vi "Format Tablet Column Span.vi"(7 "Column Count":i32=1, 11 "Spanned Cell Text":string) -> (3 "Row Text":string)   [LabVIEW 2023, in "Confluence Formatting.lvlib"]
uses:
  Confluence Formatting.lvlib
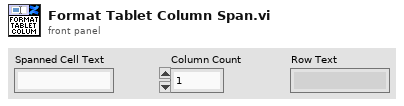
[diagram p1: front panel]
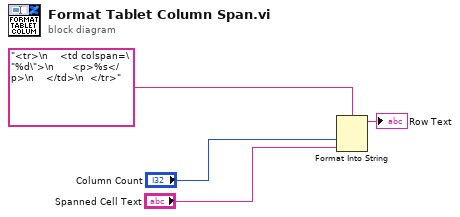
[diagram p0: block diagram]
diagram:
  n1 = Format Into String(format string="<tr>\n    <td colspan=\"%d\">\n      <p>%s</p>\n    </td>\n  </tr>", "Column Count", "Spanned Cell Text") -> (resulting string=→"Row Text":string)  [unwired: 2 in, 1 out]
